vi "PXI Sensor Inputs.vi"(2 "error in":errorcluster, 3 "Enum":T1(ring)) -> (0 "error out":errorcluster, 1 "State":bool)   [LabVIEW 2014]
uses:
  <vilib>/DAQmx/read.llb/DAQmx Read (Digital 1D U32 NChan 1Samp).vi
  <vilib>/DAQmx/miscellaneous.llb/DAQmx Fill In Error Info.vi
panel:
  out "data":u32[](array[numeric]) format="%08b"
  out "task out":refnum<k21>
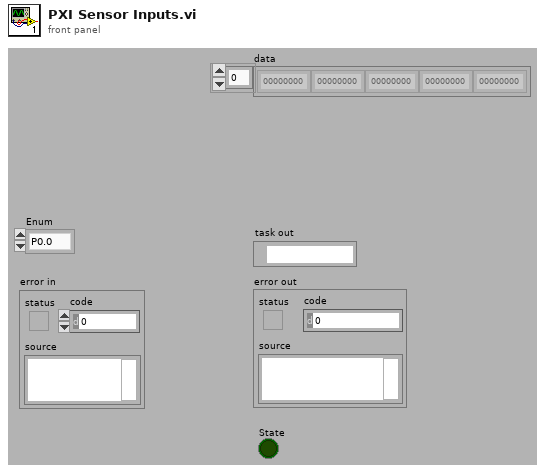
[diagram p1: front panel]
types:
  T1 = enum16{"P0.0", "P0.1", "P0.2", "P0.3", "P0.4", "P0.5", "P0.6", "P0.7", "P1.0", "P1.1", "P1.2", "P1.3", "P1.4", "P1.5", "P1.6", "P1.7", "P2.0", "P2.1", "P2.2", "P2.3", "P2.4", "P2.5", "P2.6", "P2.7", "P3.0", "P3.1", "P3.2", "P3.3", "P3.4", "P3.5", "P3.6", "P3.7", "Init", "DeInit"}
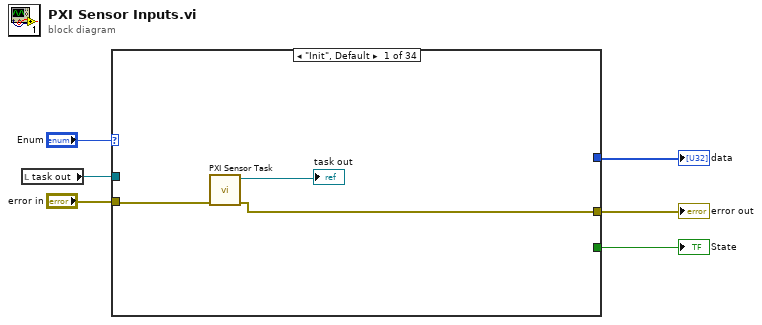
[diagram p0: block diagram]
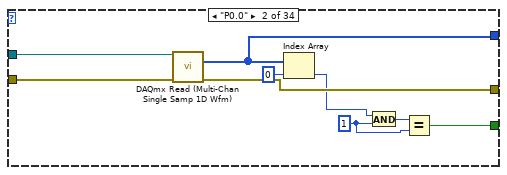
[diagram p2: hidden frame]
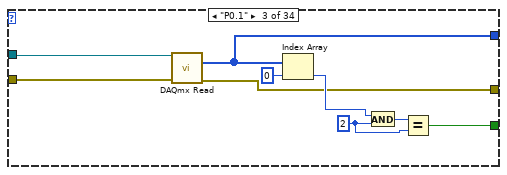
[diagram p3: hidden frame]
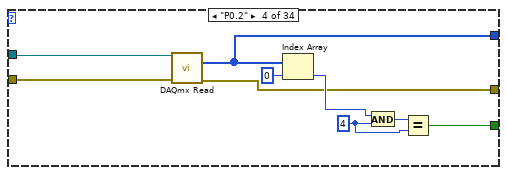
[diagram p4: hidden frame]
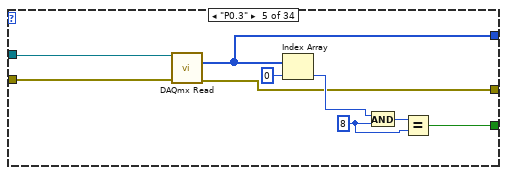
[diagram p5: hidden frame]
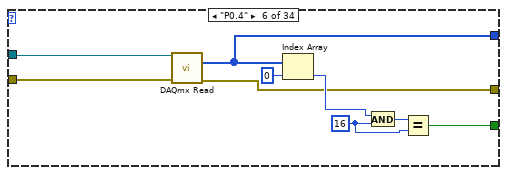
[diagram p6: hidden frame]
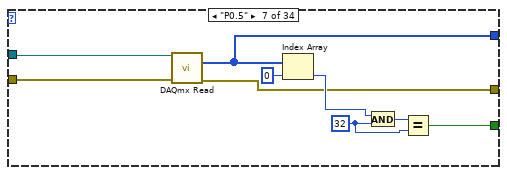
[diagram p7: hidden frame]
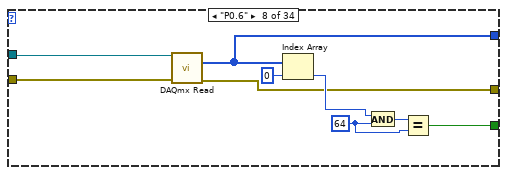
[diagram p8: hidden frame]
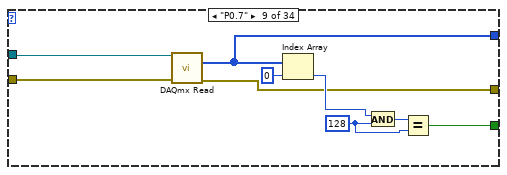
[diagram p9: hidden frame]
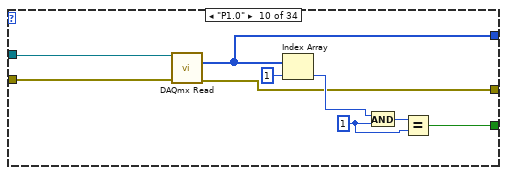
[diagram p10: hidden frame]
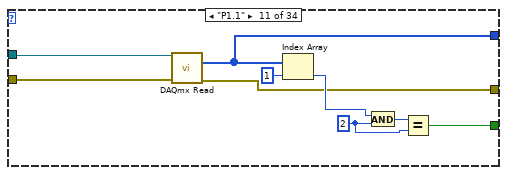
[diagram p11: hidden frame]
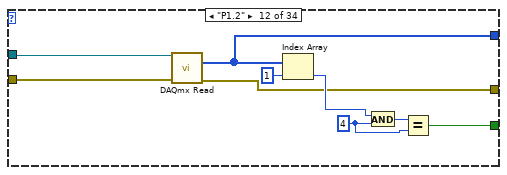
[diagram p12: hidden frame]
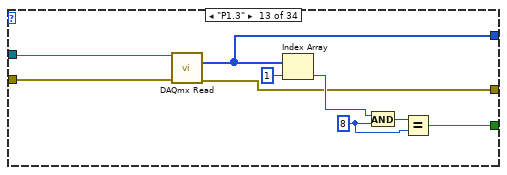
[diagram p13: hidden frame]
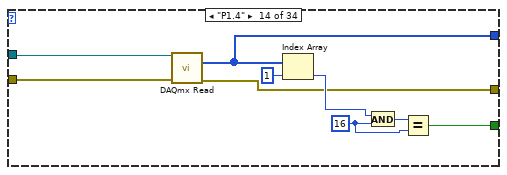
[diagram p14: hidden frame]
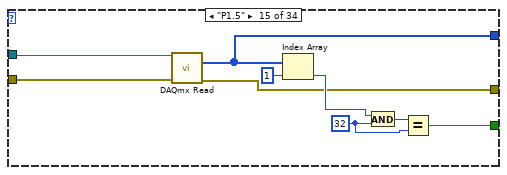
[diagram p15: hidden frame]
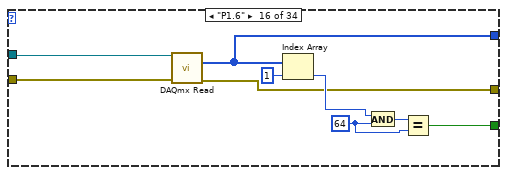
[diagram p16: hidden frame]
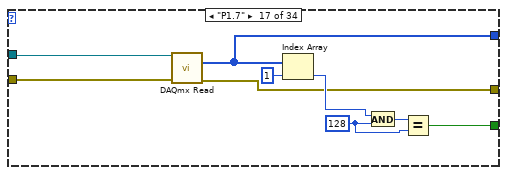
[diagram p17: hidden frame]
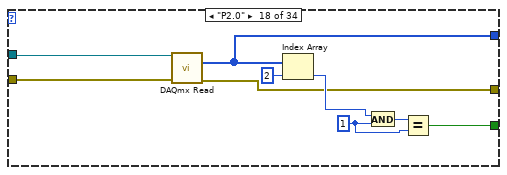
[diagram p18: hidden frame]
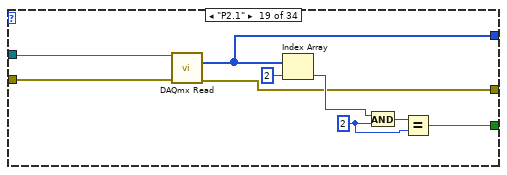
[diagram p19: hidden frame]
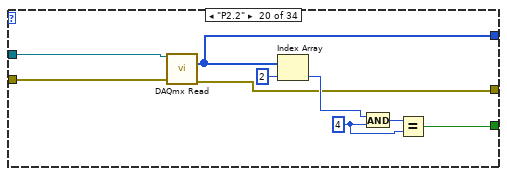
[diagram p20: hidden frame]
diagram:
  n1 = local read "task out"() -> (w4:refnum<k21>)
  n2 = case shown="\"Init\", Default" "Enum" {
    tunnel: "error in" -> [w7 w17 w23 w32 w41 w50 w59 w68 w77 w86 w95 w104 w113 w122 w131 w140 w149 w158 w167 w172 w185 w194 w203 w212 w221 w230 w239 w248 w257 w266 w275 w284 w293 w300]
    tunnel: w4 -> [_ w18 w22 w31 w40 w49 w58 w67 w76 w85 w94 w103 w112 w121 w130 w139 w148 w157 w166 w173 w184 w193 w202 w211 w220 w229 w238 w247 w256 w265 w274 w283 w292 w299]
    tunnel: [w8 w16 w21 w30 w39 w48 w57 w66 w75 w84 w93 w102 w111 w120 w129 w138 w147 w156 w165 w176 w183 w192 w201 w210 w219 w228 w237 w246 w255 w264 w273 w282 w291 w298] -> w3
    tunnel: [_ w12 w20 w29 w38 w47 w56 w65 w74 w83 w92 w101 w110 w119 w128 w137 w146 w155 w164 w175 w182 w191 w200 w209 w218 w227 w236 w245 w254 w263 w272 w281 w290 _] -> w2
    tunnel: [_ w10 w19 w28 w37 w46 w55 w64 w73 w82 w91 w100 w109 w118 w127 w136 w145 w154 w163 w174 w181 w190 w199 w208 w217 w226 w235 w244 w253 w262 w271 w280 w289 _] -> w1
    frame "Init", Default {
      n3 = call "PXI Sensor Task.vi"("error in"=w7) -> ("error out"=w8:errorcluster, "task out"=→"task out":refnum<k21>)  [unwired: 9 in]
    }
    frame "P0.0" {
      w11 = u32 1 ("y")
      n4 = call-poly "DAQmx Read (Multi-Chan Single Samp 1D Wfm).vi"("task/channels in"=w18, "error in"=w17) -> ("data"=w10:u32[], "error out"=w16:errorcluster)  [unwired: 11 in, 1 out]
      n5 = Index Array(array=w10, index=0) -> (element=w14:u32)
      n6 = And(x=w14, y=w11) -> (x .and. y?=w13:u32)
      n7 = Equal?(x=w13, y=w11) -> (x = y?=w12:bool)
    }
    frame "P0.1" {
      w24 = u32 2 ("y")
      n8 = call-poly <vilib>:"DAQmx Read.vi"("task/channels in"=w22, "error in"=w23) -> ("data"=w19:u32[], "error out"=w21:errorcluster)  [unwired: 11 in, 1 out]
      n9 = Index Array(array=w19, index=0) -> (element=w26:u32)
      n10 = And(x=w26, y=w24) -> (x .and. y?=w25:u32)
      n11 = Equal?(x=w25, y=w24) -> (x = y?=w20:bool)
    }
    frame "P0.2" {
      w33 = u32 4 ("y")
      n12 = call-poly <vilib>:"DAQmx Read.vi"("task/channels in"=w31, "error in"=w32) -> ("data"=w28:u32[], "error out"=w30:errorcluster)  [unwired: 11 in, 1 out]
      n13 = Index Array(array=w28, index=0) -> (element=w35:u32)
      n14 = And(x=w35, y=w33) -> (x .and. y?=w34:u32)
      n15 = Equal?(x=w34, y=w33) -> (x = y?=w29:bool)
    }
    frame "P0.3" {
      w42 = u32 8 ("y")
      n16 = call-poly <vilib>:"DAQmx Read.vi"("task/channels in"=w40, "error in"=w41) -> ("data"=w37:u32[], "error out"=w39:errorcluster)  [unwired: 11 in, 1 out]
      n17 = Index Array(array=w37, index=0) -> (element=w44:u32)
      n18 = And(x=w44, y=w42) -> (x .and. y?=w43:u32)
      n19 = Equal?(x=w43, y=w42) -> (x = y?=w38:bool)
    }
    frame "P0.4" {
      w51 = u32 16 ("y")
      n20 = call-poly <vilib>:"DAQmx Read.vi"("task/channels in"=w49, "error in"=w50) -> ("data"=w46:u32[], "error out"=w48:errorcluster)  [unwired: 11 in, 1 out]
      n21 = Index Array(array=w46, index=0) -> (element=w53:u32)
      n22 = And(x=w53, y=w51) -> (x .and. y?=w52:u32)
      n23 = Equal?(x=w52, y=w51) -> (x = y?=w47:bool)
    }
    frame "P0.5" {
      w60 = u32 32 ("y")
      n24 = call-poly <vilib>:"DAQmx Read.vi"("task/channels in"=w58, "error in"=w59) -> ("data"=w55:u32[], "error out"=w57:errorcluster)  [unwired: 11 in, 1 out]
      n25 = Index Array(array=w55, index=0) -> (element=w62:u32)
      n26 = And(x=w62, y=w60) -> (x .and. y?=w61:u32)
      n27 = Equal?(x=w61, y=w60) -> (x = y?=w56:bool)
    }
    frame "P0.6" {
      w69 = u32 64 ("y")
      n28 = call-poly <vilib>:"DAQmx Read.vi"("task/channels in"=w67, "error in"=w68) -> ("data"=w64:u32[], "error out"=w66:errorcluster)  [unwired: 11 in, 1 out]
      n29 = Index Array(array=w64, index=0) -> (element=w71:u32)
      n30 = And(x=w71, y=w69) -> (x .and. y?=w70:u32)
      n31 = Equal?(x=w70, y=w69) -> (x = y?=w65:bool)
    }
    frame "P0.7" {
      w78 = u32 128 ("y")
      n32 = call-poly <vilib>:"DAQmx Read.vi"("task/channels in"=w76, "error in"=w77) -> ("data"=w73:u32[], "error out"=w75:errorcluster)  [unwired: 11 in, 1 out]
      n33 = Index Array(array=w73, index=0) -> (element=w80:u32)
      n34 = And(x=w80, y=w78) -> (x .and. y?=w79:u32)
      n35 = Equal?(x=w79, y=w78) -> (x = y?=w74:bool)
    }
    frame "P1.0" {
      w87 = u32 1 ("y")
      n36 = call-poly <vilib>:"DAQmx Read.vi"("task/channels in"=w85, "error in"=w86) -> ("data"=w82:u32[], "error out"=w84:errorcluster)  [unwired: 11 in, 1 out]
      n37 = Index Array(array=w82, index=1) -> (element=w89:u32)
      n38 = And(x=w89, y=w87) -> (x .and. y?=w88:u32)
      n39 = Equal?(x=w88, y=w87) -> (x = y?=w83:bool)
    }
    frame "P1.1" {
      w96 = u32 2 ("y")
      n40 = call-poly <vilib>:"DAQmx Read.vi"("task/channels in"=w94, "error in"=w95) -> ("data"=w91:u32[], "error out"=w93:errorcluster)  [unwired: 11 in, 1 out]
      n41 = Index Array(array=w91, index=1) -> (element=w98:u32)
      n42 = And(x=w98, y=w96) -> (x .and. y?=w97:u32)
      n43 = Equal?(x=w97, y=w96) -> (x = y?=w92:bool)
    }
    frame "P1.2" {
      w105 = u32 4 ("y")
      n44 = call-poly <vilib>:"DAQmx Read.vi"("task/channels in"=w103, "error in"=w104) -> ("data"=w100:u32[], "error out"=w102:errorcluster)  [unwired: 11 in, 1 out]
      n45 = Index Array(array=w100, index=1) -> (element=w107:u32)
      n46 = And(x=w107, y=w105) -> (x .and. y?=w106:u32)
      n47 = Equal?(x=w106, y=w105) -> (x = y?=w101:bool)
    }
    frame "P1.3" {
      w114 = u32 8 ("y")
      n48 = call-poly <vilib>:"DAQmx Read.vi"("task/channels in"=w112, "error in"=w113) -> ("data"=w109:u32[], "error out"=w111:errorcluster)  [unwired: 11 in, 1 out]
      n49 = Index Array(array=w109, index=1) -> (element=w116:u32)
      n50 = And(x=w116, y=w114) -> (x .and. y?=w115:u32)
      n51 = Equal?(x=w115, y=w114) -> (x = y?=w110:bool)
    }
    frame "P1.4" {
      w123 = u32 16 ("y")
      n52 = call-poly <vilib>:"DAQmx Read.vi"("task/channels in"=w121, "error in"=w122) -> ("data"=w118:u32[], "error out"=w120:errorcluster)  [unwired: 11 in, 1 out]
      n53 = Index Array(array=w118, index=1) -> (element=w125:u32)
      n54 = And(x=w125, y=w123) -> (x .and. y?=w124:u32)
      n55 = Equal?(x=w124, y=w123) -> (x = y?=w119:bool)
    }
    frame "P1.5" {
      w132 = u32 32 ("y")
      n56 = call-poly <vilib>:"DAQmx Read.vi"("task/channels in"=w130, "error in"=w131) -> ("data"=w127:u32[], "error out"=w129:errorcluster)  [unwired: 11 in, 1 out]
      n57 = Index Array(array=w127, index=1) -> (element=w134:u32)
      n58 = And(x=w134, y=w132) -> (x .and. y?=w133:u32)
      n59 = Equal?(x=w133, y=w132) -> (x = y?=w128:bool)
    }
    frame "P1.6" {
      w141 = u32 64 ("y")
      n60 = call-poly <vilib>:"DAQmx Read.vi"("task/channels in"=w139, "error in"=w140) -> ("data"=w136:u32[], "error out"=w138:errorcluster)  [unwired: 11 in, 1 out]
      n61 = Index Array(array=w136, index=1) -> (element=w143:u32)
      n62 = And(x=w143, y=w141) -> (x .and. y?=w142:u32)
      n63 = Equal?(x=w142, y=w141) -> (x = y?=w137:bool)
    }
    frame "P1.7" {
      w150 = u32 128 ("y")
      n64 = call-poly <vilib>:"DAQmx Read.vi"("task/channels in"=w148, "error in"=w149) -> ("data"=w145:u32[], "error out"=w147:errorcluster)  [unwired: 11 in, 1 out]
      n65 = Index Array(array=w145, index=1) -> (element=w152:u32)
      n66 = And(x=w152, y=w150) -> (x .and. y?=w151:u32)
      n67 = Equal?(x=w151, y=w150) -> (x = y?=w146:bool)
    }
    frame "P2.0" {
      w159 = u32 1 ("y")
      n68 = call-poly <vilib>:"DAQmx Read.vi"("task/channels in"=w157, "error in"=w158) -> ("data"=w154:u32[], "error out"=w156:errorcluster)  [unwired: 11 in, 1 out]
      n69 = Index Array(array=w154, index=2) -> (element=w161:u32)
      n70 = And(x=w161, y=w159) -> (x .and. y?=w160:u32)
      n71 = Equal?(x=w160, y=w159) -> (x = y?=w155:bool)
    }
    frame "P2.1" {
      w168 = u32 2 ("y")
      n72 = call-poly <vilib>:"DAQmx Read.vi"("task/channels in"=w166, "error in"=w167) -> ("data"=w163:u32[], "error out"=w165:errorcluster)  [unwired: 11 in, 1 out]
      n73 = Index Array(array=w163, index=2) -> (element=w170:u32)
      n74 = And(x=w170, y=w168) -> (x .and. y?=w169:u32)
      n75 = Equal?(x=w169, y=w168) -> (x = y?=w164:bool)
    }
    frame "P2.2" {
      w180 = u32 4 ("y")
      n76 = call-poly <vilib>:"DAQmx Read.vi"("task/channels in"=w173, "error in"=w172) -> ("data"=w174:u32[], "error out"=w176:errorcluster)  [unwired: 11 in, 1 out]
      n77 = Index Array(array=w174, index=2) -> (element=w178:u32)
      n78 = And(x=w178, y=w180) -> (x .and. y?=w179:u32)
      n79 = Equal?(x=w179, y=w180) -> (x = y?=w175:bool)
    }
    frame "P2.3" {
      w186 = u32 8 ("y")
      n80 = call-poly <vilib>:"DAQmx Read.vi"("task/channels in"=w184, "error in"=w185) -> ("data"=w181:u32[], "error out"=w183:errorcluster)  [unwired: 11 in, 1 out]
      n81 = Index Array(array=w181, index=2) -> (element=w188:u32)
      n82 = And(x=w188, y=w186) -> (x .and. y?=w187:u32)
      n83 = Equal?(x=w187, y=w186) -> (x = y?=w182:bool)
    }
    frame "P2.4" {
      w195 = u32 16 ("y")
      n84 = call-poly <vilib>:"DAQmx Read.vi"("task/channels in"=w193, "error in"=w194) -> ("data"=w190:u32[], "error out"=w192:errorcluster)  [unwired: 11 in, 1 out]
      n85 = Index Array(array=w190, index=2) -> (element=w197:u32)
      n86 = And(x=w197, y=w195) -> (x .and. y?=w196:u32)
      n87 = Equal?(x=w196, y=w195) -> (x = y?=w191:bool)
    }
    frame "P2.5" {
      w204 = u32 32 ("y")
      n88 = call-poly <vilib>:"DAQmx Read.vi"("task/channels in"=w202, "error in"=w203) -> ("data"=w199:u32[], "error out"=w201:errorcluster)  [unwired: 11 in, 1 out]
      n89 = Index Array(array=w199, index=2) -> (element=w206:u32)
      n90 = And(x=w206, y=w204) -> (x .and. y?=w205:u32)
      n91 = Equal?(x=w205, y=w204) -> (x = y?=w200:bool)
    }
    frame "P2.6" {
      w213 = u32 64 ("y")
      n92 = call-poly <vilib>:"DAQmx Read.vi"("task/channels in"=w211, "error in"=w212) -> ("data"=w208:u32[], "error out"=w210:errorcluster)  [unwired: 11 in, 1 out]
      n93 = Index Array(array=w208, index=2) -> (element=w215:u32)
      n94 = And(x=w215, y=w213) -> (x .and. y?=w214:u32)
      n95 = Equal?(x=w214, y=w213) -> (x = y?=w209:bool)
    }
    frame "P2.7" {
      w222 = u32 128 ("y")
      n96 = call-poly <vilib>:"DAQmx Read.vi"("task/channels in"=w220, "error in"=w221) -> ("data"=w217:u32[], "error out"=w219:errorcluster)  [unwired: 11 in, 1 out]
      n97 = Index Array(array=w217, index=2) -> (element=w224:u32)
      n98 = And(x=w224, y=w222) -> (x .and. y?=w223:u32)
      n99 = Equal?(x=w223, y=w222) -> (x = y?=w218:bool)
    }
    frame "P3.0" {
      w231 = u32 1 ("y")
      n100 = call-poly <vilib>:"DAQmx Read.vi"("task/channels in"=w229, "error in"=w230) -> ("data"=w226:u32[], "error out"=w228:errorcluster)  [unwired: 11 in, 1 out]
      n101 = Index Array(array=w226, index=3) -> (element=w233:u32)
      n102 = And(x=w233, y=w231) -> (x .and. y?=w232:u32)
      n103 = Equal?(x=w232, y=w231) -> (x = y?=w227:bool)
    }
    frame "P3.1" {
      w240 = u32 2 ("y")
      n104 = call-poly <vilib>:"DAQmx Read.vi"("task/channels in"=w238, "error in"=w239) -> ("data"=w235:u32[], "error out"=w237:errorcluster)  [unwired: 11 in, 1 out]
      n105 = Index Array(array=w235, index=3) -> (element=w242:u32)
      n106 = And(x=w242, y=w240) -> (x .and. y?=w241:u32)
      n107 = Equal?(x=w241, y=w240) -> (x = y?=w236:bool)
    }
    frame "P3.2" {
      w249 = u32 4 ("y")
      n108 = call-poly <vilib>:"DAQmx Read.vi"("task/channels in"=w247, "error in"=w248) -> ("data"=w244:u32[], "error out"=w246:errorcluster)  [unwired: 11 in, 1 out]
      n109 = Index Array(array=w244, index=3) -> (element=w251:u32)
      n110 = And(x=w251, y=w249) -> (x .and. y?=w250:u32)
      n111 = Equal?(x=w250, y=w249) -> (x = y?=w245:bool)
    }
    frame "P3.3" {
      w258 = u32 8 ("y")
      n112 = call-poly <vilib>:"DAQmx Read.vi"("task/channels in"=w256, "error in"=w257) -> ("data"=w253:u32[], "error out"=w255:errorcluster)  [unwired: 11 in, 1 out]
      n113 = Index Array(array=w253, index=3) -> (element=w260:u32)
      n114 = And(x=w260, y=w258) -> (x .and. y?=w259:u32)
      n115 = Equal?(x=w259, y=w258) -> (x = y?=w254:bool)
    }
    frame "P3.4" {
      w267 = u32 16 ("y")
      n116 = call-poly <vilib>:"DAQmx Read.vi"("task/channels in"=w265, "error in"=w266) -> ("data"=w262:u32[], "error out"=w264:errorcluster)  [unwired: 11 in, 1 out]
      n117 = Index Array(array=w262, index=3) -> (element=w269:u32)
      n118 = And(x=w269, y=w267) -> (x .and. y?=w268:u32)
      n119 = Equal?(x=w268, y=w267) -> (x = y?=w263:bool)
    }
    frame "P3.5" {
      w276 = u32 32 ("y")
      n120 = call-poly <vilib>:"DAQmx Read.vi"("task/channels in"=w274, "error in"=w275) -> ("data"=w271:u32[], "error out"=w273:errorcluster)  [unwired: 11 in, 1 out]
      n121 = Index Array(array=w271, index=3) -> (element=w278:u32)
      n122 = And(x=w278, y=w276) -> (x .and. y?=w277:u32)
      n123 = Equal?(x=w277, y=w276) -> (x = y?=w272:bool)
    }
    frame "P3.6" {
      w285 = u32 64 ("y")
      n124 = call-poly <vilib>:"DAQmx Read.vi"("task/channels in"=w283, "error in"=w284) -> ("data"=w280:u32[], "error out"=w282:errorcluster)  [unwired: 11 in, 1 out]
      n125 = Index Array(array=w280, index=3) -> (element=w287:u32)
      n126 = And(x=w287, y=w285) -> (x .and. y?=w286:u32)
      n127 = Equal?(x=w286, y=w285) -> (x = y?=w281:bool)
    }
    frame "P3.7" {
      w294 = u32 128 ("y")
      n128 = call-poly <vilib>:"DAQmx Read.vi"("task/channels in"=w292, "error in"=w293) -> ("data"=w289:u32[], "error out"=w291:errorcluster)  [unwired: 11 in, 1 out]
      n129 = Index Array(array=w289, index=3) -> (element=w296:u32)
      n130 = And(x=w296, y=w294) -> (x .and. y?=w295:u32)
      n131 = Equal?(x=w295, y=w294) -> (x = y?=w290:bool)
    }
    frame "DeInit" {
      n132 = call <vilib>:"DAQmx Clear Task.vi"("task in"=w299, "error in"=w300) -> ("error out"=w298:errorcluster)  [unwired: 13 in]
    }
  }
  "error out" <- w3
  "State" <- w2
  "data" <- w1
